vi "S2C_UNITHERM_Poly_Initialize.vi"(8 "Error In":errorcluster, 10 "Initialize":T2={"Resource Name"="COM4", "Baud Rate"=57600, "Data Bits"=8, "Parity"=0, "Stop Bits"=10, "Flow Control"=0, "Termination Char"=10, "Enable Termination"=TRUE, "Timeout"=5000} {"Parity" items=["None", "Odd", "Even", "Mark", "Space"]; "Stop Bits" items=["1.0"=10, "1.5"=15, "2.0"=20]; "Flow Control" items=["None", "XON/XOFF", "RTS/CTS", "XON/XOFF & RTS/CTS", "DTR/DSR", "XON/XOFF & DTR/DSR"]}, 11 "Settings":T1={"Driver"="UniTherm", "Command"="Initialize", "Return"="ErrorStatus", "Parameters"="", "Timeout"=10.0}) -> (0 "Error Out":errorcluster, 3 "Response":string)   [LabVIEW 2015]
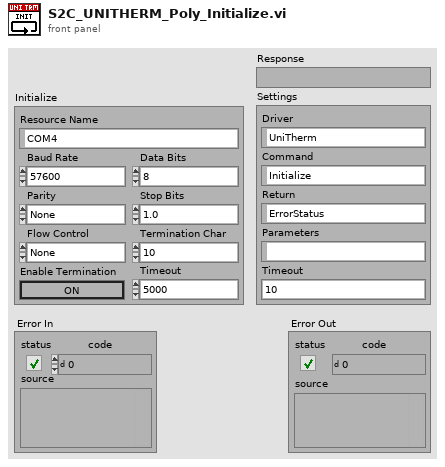
[diagram p1: front panel]
types:
  T1 = cluster{"Driver":string, "Command":string, "Return":string, "Parameters":string, "Timeout":dbl}
  T2 = cluster{"Resource Name":string, "Baud Rate":u32, "Data Bits":u16, "Parity":u16, "Stop Bits":u16, "Flow Control":u16, "Termination Char":u8, "Enable Termination":bool, "Timeout":u32}
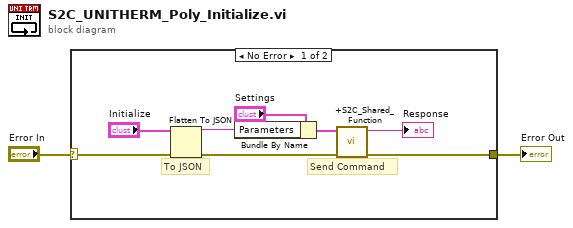
[diagram p0: block diagram]
diagram:
  n1 = case shown="No Error" "Error In" {
    selector: "Error In" -> [w5 w11]
    tunnel: [w4 w11] -> w1
    frame No Error {
      # "To JSON"
      # "Send Command"
      n2 = Flatten To JSON(anything="Initialize", error in (no error)=w5) -> (JSON string=w6:string, 11:w9:errorcluster)  [unwired: 1 in]
      n3 = Bundle By Name(cluster="Settings", "Parameters"=w6) -> (w10:T1)
      n4 = call "+S2C_Shared_Function.vi"("Error In"=w9, "Settings"=w10) -> ("Error Out"=w4:errorcluster, "Response"=→"Response":string)  [unwired: 8 in]
    }
    frame Error {
    }
  }
  "Error Out" <- w1
